vi "New Simple Adder.vi"() -> ()   [LabVIEW 2020]
panel:
  out "x+y":dbl
  in  "Numeric 2":dbl
  in  "Numeric":dbl
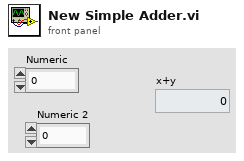
[diagram p1: front panel]
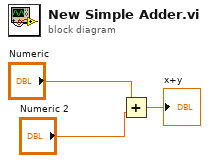
[diagram p0: block diagram]
diagram:
  n1 = Add(x="Numeric", y="Numeric 2") -> (x+y=→"x+y":dbl)
